vi "Shifter-Main.vi"() -> ()   [LabVIEW 2016]
uses:
  Shifter-state.ctl
  Shifter-control.ctl
  <vilib>/Analysis/baseanly.llb/Mean (DBL).vi
  <vilib>/Analysis/NI_AALBase.lvlib
panel:
  out "Shift state out":T1
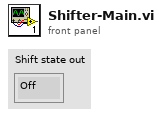
[diagram p1: front panel]
types:
  T1 = typedef "Shifter-state.ctl" = enum16{"Off", "On"}
  T2 = typedef "Shifter-control.ctl" = enum16{"Wait", "Low", "High"}
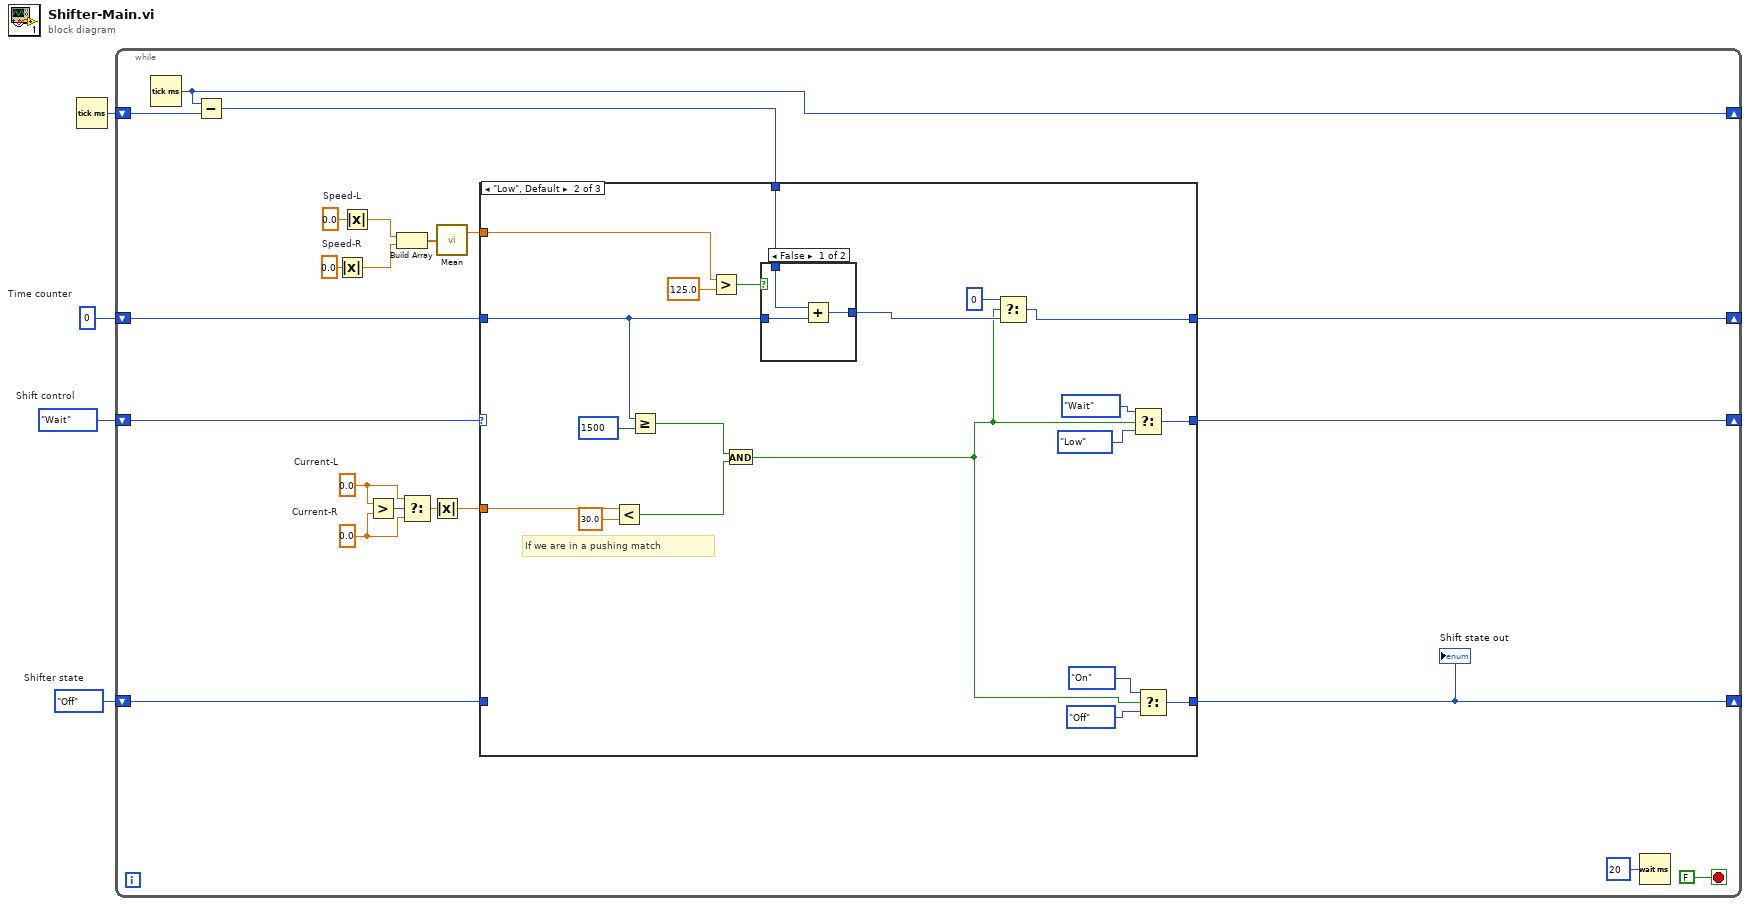
[diagram p0: block diagram]
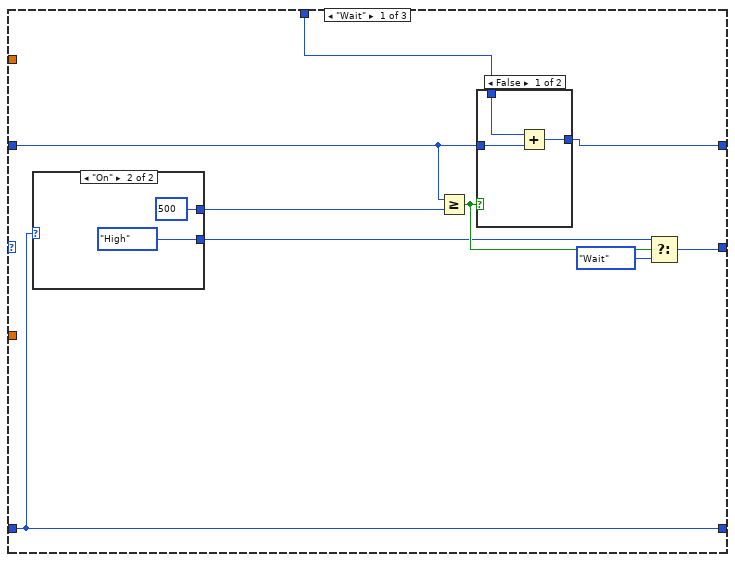
[diagram p2: hidden frame]
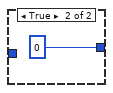
[diagram p3: hidden frame]
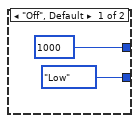
[diagram p4: hidden frame]
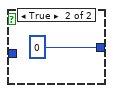
[diagram p5: hidden frame]
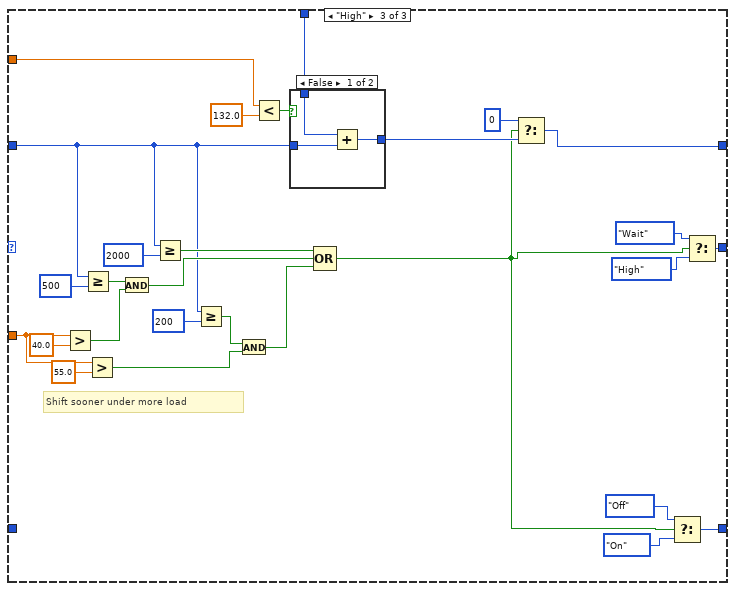
[diagram p6: hidden frame]
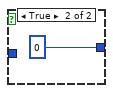
[diagram p7: hidden frame]
diagram:
  w1 = Shifter-state."Off"  # Shifter state
  w2 = Shifter-control."Wait"  # Shift control
  w3 = u32 0  # Time counter
  n1 = Tick Count (ms)() -> (millisecond timer value=w4:u32)
  n2 = while {
    shift-right: [w23] -> _
    shift-left: w4 -> [w24]
    shift-right: [w20] -> _
    shift-left: w3 -> [w19]
    shift-right: [w10] -> _
    shift-left: w1 -> [w11]
    shift-right: [w9] -> _
    shift-left: w2 -> [w17]
    stop <- FALSE stop-if-true
    w6 = 0.0  # Current-R
    w15 = 0.0  # Speed-R
    w16 = 0.0  # Speed-L
    w7 = 0.0  # Current-L
    n3 = Tick Count (ms)() -> (millisecond timer value=w23:u32)
    n4 = Subtract(x=w23, y=w24) -> (x-y=w21:u32)
    n5 = Absolute Value(x=w15) -> ()  [unwired: 1 out]
    n6 = Absolute Value(x=w16) -> (abs(x)=w14:dbl)
    n7 = Greater?(x=w7, y=w6) -> (0:w8:bool)
    n8 = Build Array(w14, w15) -> (w13:dbl[])
    n9 = Select(t=w7, s=w8, f=w6) -> (s? t:f=w5:dbl)
    n10 = Absolute Value(x=w5) -> (abs(x)=w18:dbl)
    n11 = call-poly <vilib>:"Mean.vi"("X"=w13) -> ("mean"=w12:dbl)  [unwired: 1 out]
    n12 = case shown="\"Low\", Default" w17 {
      tunnel: w21 -> [w33 w62 w94]
      tunnel: [w31 w55 w75] -> w20
      tunnel: w19 -> [w32 w59 w82]
      tunnel: w18 -> [_ w47 w88]
      tunnel: w12 -> [_ w58 w76]
      tunnel: w11 -> [w34 _ _]
      tunnel: [w34 w49 w68] -> w10
      tunnel: [w29 w48 w73] -> w9
      frame "Wait" {
        n13 = case shown="\"On\"" w34 {
          tunnel: [Shifter-control."Low" Shifter-control."High"] -> w27
          tunnel: [u32 1000 u32 500] -> w30
          frame "Off", Default {
          }
          frame "On" {
          }
        }
        n14 = Greater Or Equal?(x=w32, y=w30) -> (x >= y?=w28:bool)
        n15 = case shown="False" w28 {
          tunnel: w32 -> [w37 _]
          tunnel: w33 -> [w36 _]
          tunnel: [w35 u32 0] -> w31
          frame False {
            n16 = Add(x=w36, y=w37) -> (x+y=w35:u32)
          }
          frame True {
          }
        }
        n17 = Select(t=w27, s=w28, f=Shifter-control."Wait") -> (s? t:f=w29:T2)
      }
      frame "Low", Default {
        # "If we are in a pushing match"
        n18 = Less?(x=w47, y=30.0) -> (x < y?=w44:bool)
        n19 = Greater Or Equal?(x=w59, y=u32 1500) -> (x >= y?=w45:bool)
        n20 = Greater?(x=w58, y=125.0) -> (0:w57:bool)
        n21 = And(x=w45, y=w44) -> (x .and. y?=w43:bool)
        n22 = case shown="False" w57 {
          tunnel: w59 -> [w65 _]
          tunnel: w62 -> [w64 _]
          tunnel: [w63 u32 0] -> w61
          frame False {
            n23 = Add(x=w64, y=w65) -> (x+y=w63:u32)
          }
          frame True {
          }
        }
        n24 = Select(t=u32 0, s=w43, f=w61) -> (s? t:f=w55:u32)
        n25 = Select(t=Shifter-control."Wait", s=w43, f=Shifter-control."Low") -> (s? t:f=w48:T2)
        n26 = Select(t=Shifter-state."On", s=w43, f=Shifter-state."Off") -> (s? t:f=w49:T1)
      }
      frame "High" {
        # "Shift sooner under more load"
        n27 = Greater?(x=w88, y=40.0) -> (0:w86:bool)
        n28 = Greater Or Equal?(x=w82, y=u32 500) -> (x >= y?=w87:bool)
        n29 = Greater?(x=w88, y=55.0) -> (0:w80:bool)
        n30 = And(x=w87, y=w86) -> (x .and. y?=w84:bool)
        n31 = Greater Or Equal?(x=w82, y=u32 2000) -> (x >= y?=w85:bool)
        n32 = Greater Or Equal?(x=w82, y=u32 200) -> (x >= y?=w81:bool)
        n33 = And(x=w81, y=w80) -> (x .and. y?=w79:bool)
        n34 = Less?(x=w76, y=132.0) -> (x < y?=w77:bool)
        n35 = case shown="False" w77 {
          tunnel: w82 -> [w97 _]
          tunnel: w94 -> [w96 _]
          tunnel: [w95 u32 0] -> w93
          frame False {
            n36 = Add(x=w96, y=w97) -> (x+y=w95:u32)
          }
          frame True {
          }
        }
        n37 = Compound Arithmetic op=OR(w85, w84, w79) -> (w67:bool)
        n38 = Select(t=u32 0, s=w67, f=w93) -> (s? t:f=w75:u32)
        n39 = Select(t=Shifter-state."Off", s=w67, f=Shifter-state."On") -> (s? t:f=w68:T1)
        n40 = Select(t=Shifter-control."Wait", s=w67, f=Shifter-control."High") -> (s? t:f=w73:T2)
      }
    }
    "Shift state out" <- w10
    n41 = Wait (ms)(milliseconds to wait=u32 20) -> ()  [unwired: 1 out]
  }
